vi "String2file.vi"(8 "Error In":errorcluster, 9 "Input String":string, 10 "FileName":string, 11 "Base Path":path) -> (0 "Error Out":errorcluster)   [LabVIEW 2020]
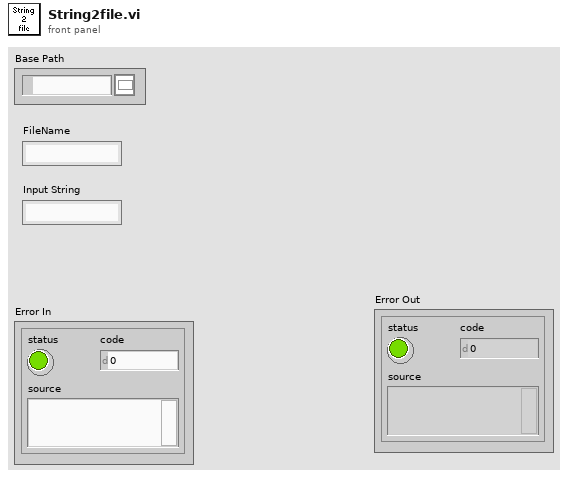
[diagram p1: front panel]
types:
  T1 = enum16{"open", "replace", "create", "open or create", "replace or create", "replace or create with confirmation"}
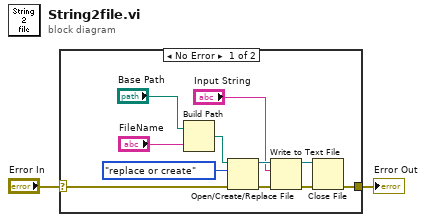
[diagram p0: block diagram]
diagram:
  n1 = case shown="No Error" "Error In" {
    selector: "Error In" -> [w4 w14]
    tunnel: [w8 w14] -> w2
    frame No Error {
      n2 = Build Path(base path="Base Path", name or relative path="FileName") -> (appended path=w11:path)
      n3 = Open/Create/Replace File(file path (use dialog)=w11, error in=w4, operation (0:open)=T1."replace or create") -> (refnum out=w12:refnum<file>, error out=w10:errorcluster)  [unwired: 3 in, 1 out]
      n4 = Write to Text File(file (use dialog)=w12, text="Input String", error in=w10) -> (refnum out=w13:refnum<file>, error out=w9:errorcluster)  [unwired: 1 in, 1 out]
      n5 = Close File(refnum=w13, error in=w9) -> (error out=w8:errorcluster)  [unwired: 1 out]
    }
    frame Error {
    }
  }
  "Error Out" <- w2
